vi "Camera Process.vi"(1 "error in":errorcluster) -> ()   [LabVIEW 2013]
uses:
  Camera Global Data.vi
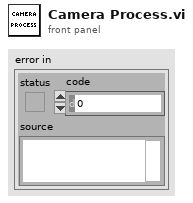
[diagram p1: front panel]
types:
  T1 = cluster{"Servo Angle Get":dbl, "Servo Angle Set":dbl}
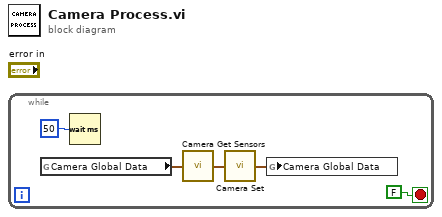
[diagram p0: block diagram]
diagram:
  n1 = while {
    stop <- FALSE stop-if-true
    n2 = global read "Camera Global Data.vi" "Camera Global Data"() -> (w3:T1)
    n3 = Wait (ms)(milliseconds to wait=u32 50) -> ()  [unwired: 1 out]
    n4 = call "Camera Get Sensors.vi"("Camera Global Data in"=w3) -> ("Camera Global Data out"=w2:T1)
    n5 = call "Camera Set.vi"("Camera Global Data in"=w2) -> ("Camera Global Data out"=w1:T1)
    n6 = global write "Camera Global Data.vi" "Camera Global Data"(w1) -> ()
  }
